vi "Erase.vi"(0 "Data":cluster{cluster{dbl, dbl}[]}[](array[cluster])) -> (14 "Data":cluster{cluster{dbl, dbl}[]}[](array[cluster]))   [LabVIEW 2018]
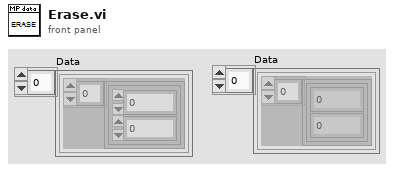
[diagram p1: front panel]
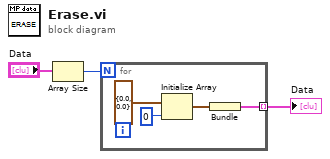
[diagram p0: block diagram]
diagram:
  n1 = Array Size(array="Data") -> (size(s)=w2:i32)
  n2 = for {
    N: w2 -> [_]
    tunnel: [w7] -> w3 mode=indexing
    n3 = Initialize Array(cluster{dbl, dbl} {0.0, 0.0}, 0 ("dimension size")) -> (w5:cluster{dbl, dbl}[])
    n4 = Bundle(w5) -> (w7:cluster{cluster{dbl, dbl}[]})  [unwired: 1 in]
  }
  "Data" <- w3
